vi "Search Array__ogtk.vi"   [LabVIEW 2016]
doc: "Searches for all element data matches in array"
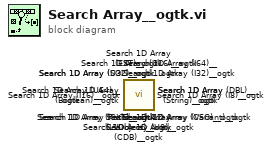
[diagram p0: block diagram]
diagram:
  n1 = call <userlib>:"Search 1D Array (LVObject)__ogtk.vi"() -> ()  [unwired: 9 in, 1 out]
  n2 = call <userlib>:"Search 1D Array (I64)__ogtk.vi"() -> ()  [unwired: 9 in, 1 out]
  n3 = call <userlib>:"Search 1D Array (U64)__ogtk.vi"() -> ()  [unwired: 9 in, 1 out]
  n4 = call <userlib>:"Search 1D Array (DBL)__ogtk.vi"() -> ()  [unwired: 9 in, 1 out]
  n5 = call <userlib>:"Search 1D Array (SGL)__ogtk.vi"() -> ()  [unwired: 9 in, 1 out]
  n6 = call <userlib>:"Search 1D Array (EXT)__ogtk.vi"() -> ()  [unwired: 9 in, 1 out]
  n7 = call <userlib>:"Search 1D Array (CSG)__ogtk.vi"() -> ()  [unwired: 9 in, 1 out]
  n8 = call <userlib>:"Search 1D Array (CDB)__ogtk.vi"() -> ()  [unwired: 9 in, 1 out]
  n9 = call <userlib>:"Search 1D Array (CXT)__ogtk.vi"() -> ()  [unwired: 9 in, 1 out]
  n10 = call <userlib>:"Search 1D Array (I8)__ogtk.vi"() -> ()  [unwired: 9 in, 1 out]
  n11 = call <userlib>:"Search 1D Array (I16)__ogtk.vi"() -> ()  [unwired: 9 in, 1 out]
  n12 = call <userlib>:"Search 1D Array (I32)__ogtk.vi"() -> ()  [unwired: 9 in, 1 out]
  n13 = call <userlib>:"Search 1D Array (U8)__ogtk.vi"() -> ()  [unwired: 9 in, 1 out]
  n14 = call <userlib>:"Search 1D Array (U16)__ogtk.vi"() -> ()  [unwired: 9 in, 1 out]
  n15 = call <userlib>:"Search 1D Array (U32)__ogtk.vi"() -> ()  [unwired: 9 in, 1 out]
  n16 = call <userlib>:"Search 1D Array (Boolean)__ogtk.vi"() -> ()  [unwired: 9 in, 1 out]
  n17 = call <userlib>:"Search 1D Array (String)__ogtk.vi"() -> ()  [unwired: 9 in, 1 out]
  n18 = call <userlib>:"Search 1D Array (Path)__ogtk.vi"() -> ()  [unwired: 9 in, 1 out]
  n19 = call <userlib>:"Search 1D Array (Variant)__ogtk.vi"() -> ()  [unwired: 9 in, 1 out]
